vi "Add gRPC Server to Map.vi"(8 "error in (no error)":errorcluster, 10 "gRPC Server Class":refnum<class "PluginCore.lvclass">, 11 "CIFTemplateNode in":refnum<class "CIFCorePlugin.lvclass">) -> (0 "error out":errorcluster, 3 "CIFTemplateNode out":refnum<class "CIFCorePlugin.lvclass">)   [LabVIEW 2021, in "CIFCorePlugin.lvclass"]
uses:
  CIFCorePlugin.lvclass
  CIFCoreGrpc/CIFCorePlugin_server/RPC Service/PluginCore/PluginCore.lvclass
  CIFCorePlugin.lvclass/CIFCorePlugin.ctl
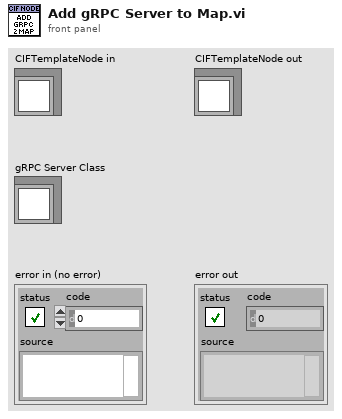
[diagram p1: front panel]
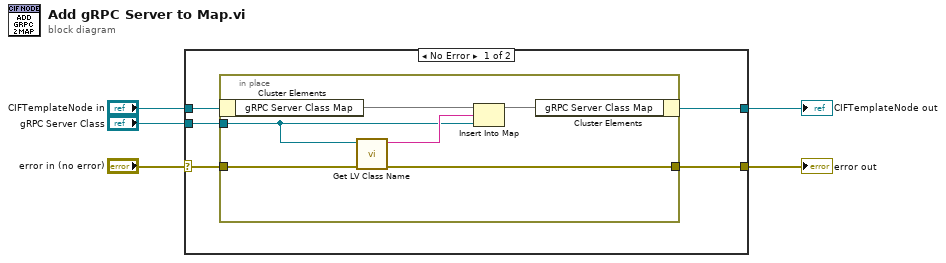
[diagram p0: block diagram]
diagram:
  n1 = case shown="No Error" "error in (no error)" {
    selector: "error in (no error)" -> [w8 w18]
    tunnel: [w7 w18] -> w4
    tunnel: [w9 w17] -> w2
    tunnel: "CIFTemplateNode in" -> [w10 w17]
    tunnel: "gRPC Server Class" -> [w6 _]
    frame No Error {
      n2 = in-place {
        in-place-border: w8 -> [w13]
        in-place-border: [w12] -> w7
        in-place-border: w6 -> [w11]
        n3 = in-place-cluster #1(w10) -> ("gRPC Server Class Map"=w16:map{string, refnum<class "PluginCore.lvclass">})
        n4 = call <vilib>:"Get LV Class Name.vi"("error in (no error)"=w13, "object"=w11) -> ("error out"=w12:errorcluster, "class name"=w14:string)  [unwired: 8 in]
        n5 = Insert Into Map(map in=w16, key=w14, value=w11) -> (map out=w15:map{string, refnum<class "PluginCore.lvclass">})  [unwired: 2 out]
        n6 = in-place-cluster #1("gRPC Server Class Map"=w15) -> (w9:refnum<class "CIFCorePlugin.lvclass">)
      }
    }
    frame Error {
    }
  }
  "error out" <- w4
  "CIFTemplateNode out" <- w2
